vi "HTML JS Template.vi"(4 "Show Border":bool=TRUE, 6 "Refresh rate (250ms)":i32=250, 8 "Synchronous Requests":bool=TRUE, 9 "Websocket Info":T1, 10 "js":T2, 11 "HTML":T3) -> (2 "js out":string, 3 "HTML out":string)   [LabVIEW 2015, in "Front Panel Publisher.lvlib" / "Web Front Panel.lvclass"]
uses:
  Web Front Panel.lvclass
  Controls/HTML Template Fill.ctl
  Controls/JS Template Fill.ctl
  Front Panel Manager_class/Controls/Websocket Info.ctl
  <vilib>/wsapi/NI_WebServices.lvlib
  Front Panel Manager_class/Front Panel Manager.lvclass
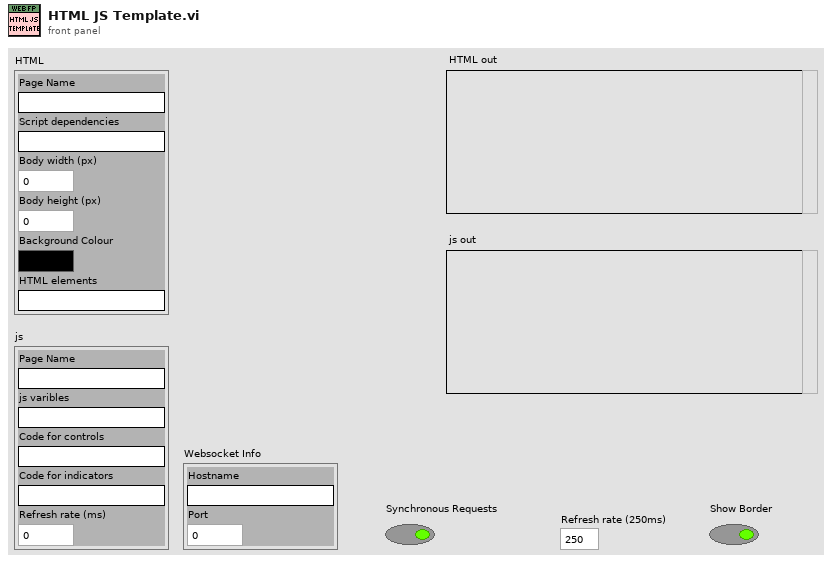
[diagram p1: front panel]
types:
  T1 = typedef "Front Panel Publisher.lvlib/Front Panel Manager.lvclass/Websocket Info.ctl" = cluster{"Hostname":string, "Port":u16}
  T2 = typedef "Front Panel Publisher.lvlib/Web Front Panel.lvclass/JS Template Fill.ctl" = cluster{"Page Name":string, "js varibles":string, "Code for controls":string, "Code for indicators":string, "Refresh rate (ms)":i32}
  T3 = typedef "Front Panel Publisher.lvlib/Web Front Panel.lvclass/HTML Template Fill.ctl" = cluster{"Page Name":string, "Script dependencies":string, "Body width (px)":i32, "Body height (px)":i32, "Background Colour":u32, "HTML elements":string}
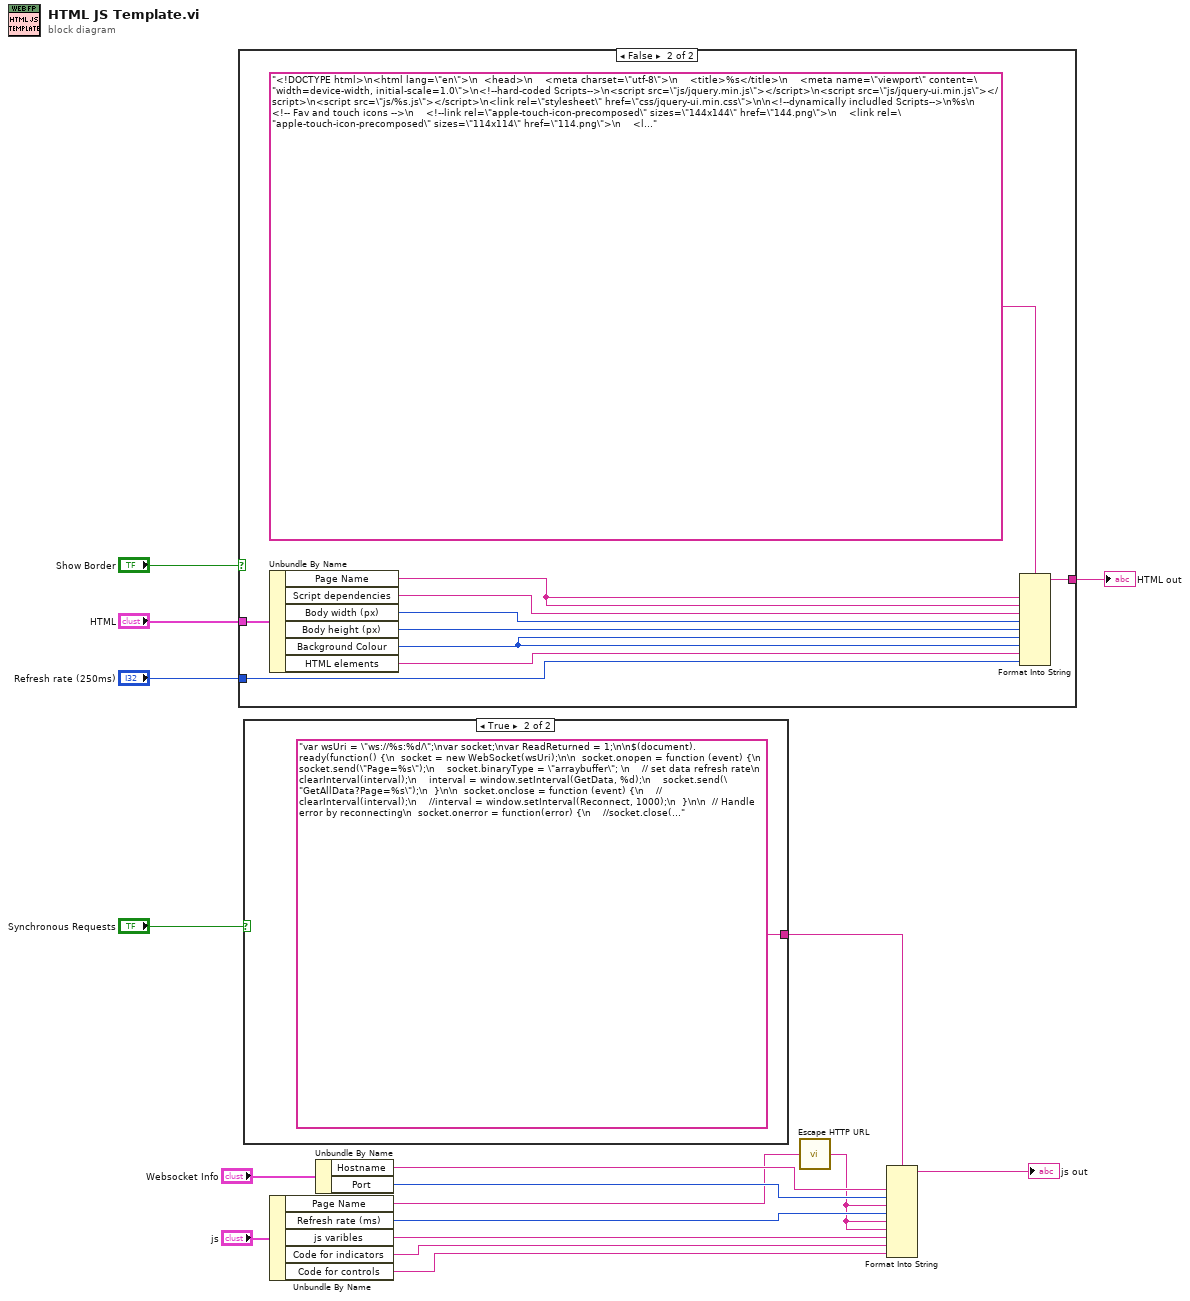
[diagram p0: block diagram]
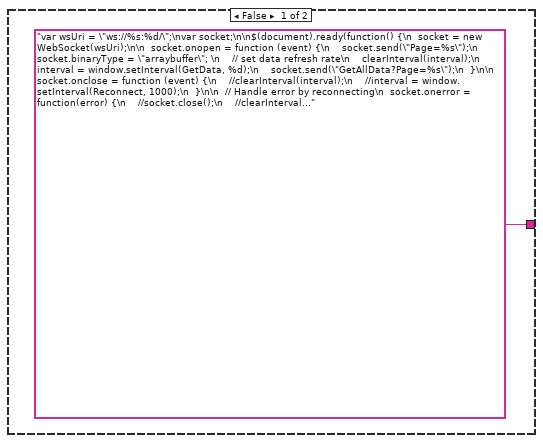
[diagram p2: hidden frame]
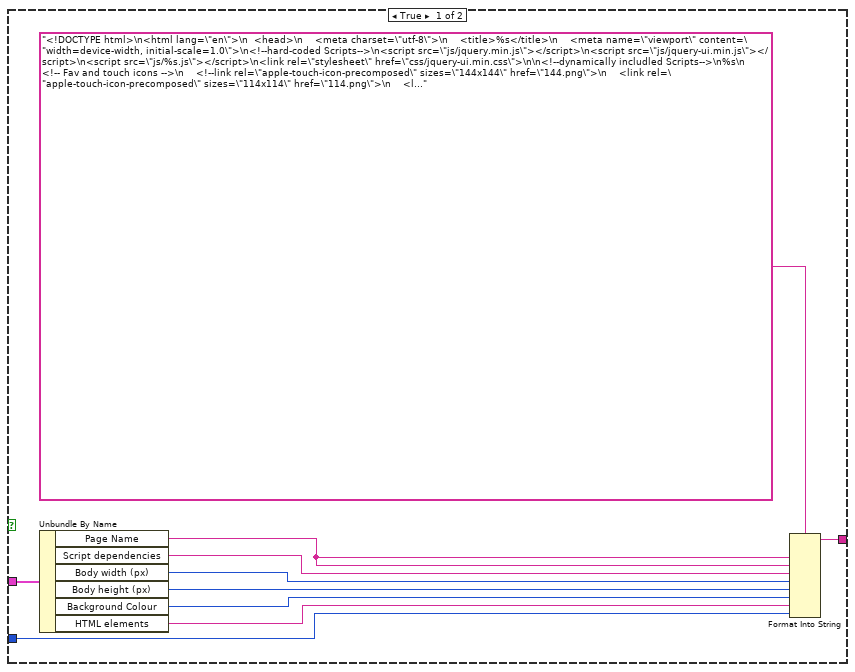
[diagram p3: hidden frame]
diagram:
  n1 = case shown="False" "Show Border" {
    tunnel: [w26 w36] -> w17
    tunnel: "HTML" -> [w25 w35]
    tunnel: "Refresh rate (250ms)" -> [w18 w29]
    frame True {
      n2 = Unbundle By Name(w25) -> ("Page Name"=w24:string, "Script dependencies"=w23:string, "Body width (px)"=w22:i32, "Body height (px)"=w21:i32, "Background Colour"=w19:u32, "HTML elements"=w20:string)
      n3 = Format Into String(format string="<!DOCTYPE html>\n<html lang=\"en\">\n  <head>\n    <meta charset=\"utf-8\">\n    <title>%s</title>\n    <meta name=\"viewport\" content=\"width=device-width, initial-scale=1.0\">\n<!--hard-coded Scripts-->\n<script src=\"js/jquery.min.js\"></script>\n<script src=\"js/jquery-ui.min.js\"></script>\n<script src=\"js/%s.js\"></script>\n<link rel=\"stylesheet\" href=\"css/jquery-ui.min.css\">\n\n<!--dynamically includled Scripts-->\n%s\n    <!-- Fav and touch icons -->\n    <!--link rel=\"apple-touch-icon-precomposed\" sizes=\"144x144\" href=\"144.png\">\n    <link rel=\"apple-touch-icon-precomposed\" sizes=\"114x114\" href=\"114.png\">\n    <link rel=\"apple-touch-icon-precomposed\" sizes=\"72x72\" href=\"72.png\">\n    <link rel=\"apple-touch-icon-precomposed\" href=\"57.png\"-->\n    <link rel=\"shortcut icon\" href=\"favicon.ico\">\n  </head>\n\n  <body style=\"position: absolute; width: %dpx; height: %dpx;border-radius: 5px; border: 1px solid #000000; background-color: #%x;\">\n%s\n  <div id=\"settingsDlg\" title=\"Settings\"><form><fieldset>\n    <label>Refresh rate (ms):</label>\n    <input type=\"text\" name=\"refreshRate\" id=\"refreshRate\" value=\"%d\" class=\"text ui-widget-content ui-corner-all\"></fieldset></form>\n  </div>\n  <img id=\"settingsBtn\" style=\"position: fixed; bottom: 0px; right: 0px;\" src=\"img/cog.png\" title=\"Settings\">\n</body>\n</html>", w24, w24, w23, w22, w21, w19, w20, w18) -> (resulting string=w26:string)  [unwired: 2 in, 1 out]
    }
    frame False {
      n4 = Unbundle By Name(w35) -> ("Page Name"=w34:string, "Script dependencies"=w33:string, "Body width (px)"=w32:i32, "Body height (px)"=w31:i32, "Background Colour"=w28:u32, "HTML elements"=w30:string)
      n5 = Format Into String(format string="<!DOCTYPE html>\n<html lang=\"en\">\n  <head>\n    <meta charset=\"utf-8\">\n    <title>%s</title>\n    <meta name=\"viewport\" content=\"width=device-width, initial-scale=1.0\">\n<!--hard-coded Scripts-->\n<script src=\"js/jquery.min.js\"></script>\n<script src=\"js/jquery-ui.min.js\"></script>\n<script src=\"js/%s.js\"></script>\n<link rel=\"stylesheet\" href=\"css/jquery-ui.min.css\">\n\n<!--dynamically includled Scripts-->\n%s\n    <!-- Fav and touch icons -->\n    <!--link rel=\"apple-touch-icon-precomposed\" sizes=\"144x144\" href=\"144.png\">\n    <link rel=\"apple-touch-icon-precomposed\" sizes=\"114x114\" href=\"114.png\">\n    <link rel=\"apple-touch-icon-precomposed\" sizes=\"72x72\" href=\"72.png\">\n    <link rel=\"apple-touch-icon-precomposed\" href=\"57.png\"-->\n    <link rel=\"shortcut icon\" href=\"favicon.ico\">\n  </head>\n\n  <body style=\"position: absolute; width: %dpx; height: %dpx;border-radius: 5px; border: 1px solid #%x; background-color: #%x;\">\n%s\n  <div id=\"settingsDlg\" title=\"Settings\"><form><fieldset>\n    <label>Refresh rate (ms):</label>\n    <input type=\"text\" name=\"refreshRate\" id=\"refreshRate\" value=\"%d\" class=\"text ui-widget-content ui-corner-all\"></fieldset></form>\n  </div>\n  <img id=\"settingsBtn\" style=\"position: fixed; bottom: 0px; right: 0px;\" src=\"img/cog.png\" title=\"Settings\">\n</body>\n</html>", w34, w34, w33, w32, w31, w28, w28, w30, w29) -> (resulting string=w36:string)  [unwired: 2 in, 1 out]
    }
  }
  "HTML out" <- w17
  n6 = case shown="True" "Synchronous Requests" {
    tunnel: ["var wsUri = \"ws://%s:%d/\";\nvar socket;\n\n$(document).ready(function() {\n  socket = new WebSocket(wsUri);\n\n  socket.onopen = function (event) {\n    socket.send(\"Page=%s\");\n    socket.binaryType = \"arraybuffer\"; \n    // set data refresh rate\n    clearInterval(interval);\n    interval = window.setInterval(GetData, %d);\n    socket.send(\"GetAllData?Page=%s\");\n  }\n\n  socket.onclose = function (event) {\n    //clearInterval(interval);\n    //interval = window.setInterval(Reconnect, 1000);\n  }\n\n  // Handle error by reconnecting\n  socket.onerror = function(error) {\n    //socket.close();\n    //clearInterval(interval);\n    //interval = window.setInterval(Reconnect, 1000);\n  }\n\n// Request new data for this page\nfunction GetData() {\n\tif (socket.readyState = 1) {\n\t\tsocket.send(\"GetData?Page=%s\");\n\t}\n};\n\n// Reconnect\nfunction Reconnect() {\n  socket = new WebSocket(wsUri);\n}\n\n// webservice stuff\nvar interval;\n\n// set up the settings dialog\nvar dialog = $( \"#settingsDlg\" );\n\ndialog = $( \"#settingsDlg\" ).dialog({\n  autoOpen: false,\n  modal: true,\n  buttons: {\n    \"OK\": function() {\n      clearInterval(interval);\n      interval = window.setInterval(GetData, $( \"#refreshRate\" ).val());\n      dialog.dialog( \"close\" );\n    },\n    Cancel: function() {\n      dialog.dialog( \"close\" );\n    }\n  }\n});\n$( \"#settingsBtn\" ).click(function() {\n  dialog.dialog( \"open\" );\n});\n\n// variables for created objects\n%s\n\n// Incoming Event Handler\nsocket.onmessage = function(msg) {\n  res = JSON.parse(msg.data);\n// object specific code to manipulate variables defined above\n%s\n}\n\n// Additional functions for controls\n%s\n});\n\n$(window).bind('beforeunload', function() {\n  socket.send(\"close\");\n  socket.close();\n});" "var wsUri = \"ws://%s:%d/\";\nvar socket;\nvar ReadReturned = 1;\n\n$(document).ready(function() {\n  socket = new WebSocket(wsUri);\n\n  socket.onopen = function (event) {\n    socket.send(\"Page=%s\");\n    socket.binaryType = \"arraybuffer\"; \n    // set data refresh rate\n    clearInterval(interval);\n    interval = window.setInterval(GetData, %d);\n    socket.send(\"GetAllData?Page=%s\");\n  }\n\n  socket.onclose = function (event) {\n    //clearInterval(interval);\n    //interval = window.setInterval(Reconnect, 1000);\n  }\n\n  // Handle error by reconnecting\n  socket.onerror = function(error) {\n    //socket.close();\n    //clearInterval(interval);\n    //interval = window.setInterval(Reconnect, 1000);\n  }\n\n// Request new data for this page\nfunction GetData() {\n\tif (socket.readyState = 1 && ReadReturned) {\n\tReadReturned = 0;\n\t\tsocket.send(\"GetData?Page=%s\");\n\t}\n};\n\n// Reconnect\nfunction Reconnect() {\n  socket = new WebSocket(wsUri);\n}\n\n// webservice stuff\nvar interval;\n\n// set up the settings dialog\nvar dialog = $( \"#settingsDlg\" );\n\ndialog = $( \"#settingsDlg\" ).dialog({\n  autoOpen: false,\n  modal: true,\n  buttons: {\n    \"OK\": function() {\n      clearInterval(interval);\n      interval = window.setInterval(GetData, $( \"#refreshRate\" ).val());\n      dialog.dialog( \"close\" );\n    },\n    Cancel: function() {\n      dialog.dialog( \"close\" );\n    }\n  }\n});\n$( \"#settingsBtn\" ).click(function() {\n  dialog.dialog( \"open\" );\n});\n\n// variables for created objects\n%s\n\n// Incoming Event Handler\nsocket.onmessage = function(msg) {\n  ReadReturned = 1;\n  res = JSON.parse(msg.data);\n// object specific code to manipulate variables defined above\n%s\n}\n\n// Additional functions for controls\n%s\n});\n\n$(window).bind('beforeunload', function() {\n  socket.send(\"close\");\n  socket.close();\n});"] -> w14
    frame False {
    }
    frame True {
    }
  }
  n7 = Unbundle By Name("js") -> ("Page Name"=w3:string, "Refresh rate (ms)"=w7:i32, "js varibles"=w6:string, "Code for indicators"=w12:string, "Code for controls"=w11:string)
  n8 = Unbundle By Name("Websocket Info") -> ("Hostname"=w8:string, "Port"=w9:u16)
  n9 = call <vilib>:"Escape HTTP URL.vi"("unescaped string in"=w3) -> ("escaped string out"=w2:string)
  n10 = Format Into String(format string=w14, w8, w9, w2, w7, w2, w2, w6, w12, w11) -> (resulting string=→"js out":string)  [unwired: 2 in, 1 out]
